vi "LIDAR Loop.vi"() -> ()   [LabVIEW 2011]
uses:
  <vilib>/Platform/TimedLoop/XDataNode/timing_clust.ctl
  <vilib>/Platform/TimedLoop/XDataNode/nitl_modes.ctl
  <vilib>/Platform/TimedLoop/XDataNode/wakeup.ctl
  <instrlib>/Hokuyo URG Series/Public/Initialize-Standard.vi
  <vilib>/Platform/TimedLoop/XDataNode/XDataNode.xnode
  <vilib>/Platform/TimedLoop/XDataNode/XDNodeRunTimeDep.lvlib
  <instrlib>/Hokuyo URG Series/Hokuyo URG Series.lvlib
panel:
  in  "maximum":dbl=300.0 format="%0.2f"
  out "Data Aquired":picture
  in  "error in":errorcluster
  in  "VISA resource name":refnum<visa-resource-name>
  in  "Debug":bool=TRUE
  out "LIDAR Data":cluster{"Magnitude":dbl[], "Direction":dbl[]}
  in  "end point (135°)":dbl=135.0
  in  "start point (-135°)":dbl=-135.0
  out "error out":errorcluster
  in  "protocol":u32(ring)=2 items=["Convert to Latest", "SCIP 1.1", "SCIP 2.0"]
  in  "stop?":bool
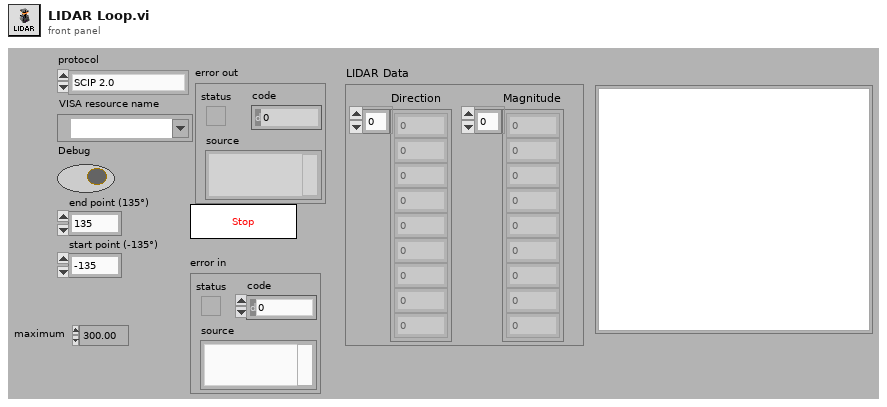
[diagram p1: front panel]
types:
  T1 = typedef "XDNodeRunTimeDep.lvlib/timing_clust.ctl" = cluster{"Expected End [f-1]":u64, "Actual End [f-1]":u64, "Finished Late? [f-1]":bool, "Expected End [i-1]":u64, "Actual End [i-1]":u64, "Finished Late? [i-1]":bool, "Expected Start [i]":u64, "Actual Start [i]":u64, "Expected Start [f]":u64, "Actual Start [f]":u64, "Source Name":string, "Structure Name":string, "Period":i64, "Deadline":i64, "Offset":i64, "Start":i64, "Priority":i32, "Timeout":i32, "Mode":T2, "Wakeup Reason":T3, "Error":errorcluster, "Source Type":string, "Secondary Source Type":string, "Global End Time":u64, "Global Start Time":u64, "Frame Duration":u64, "Iteration Duration":u64, "Assigned CPU":i32, "I/O Scan Engine Mode":u32}
  T2 = typedef "XDNodeRunTimeDep.lvlib/nitl_modes.ctl" = enum32{"No Change", "Process missed periods, maintain original phase", "Discard missed periods, maintain original phase", "Process missed periods, ignore original phase", "Discard missed periods, ignore original phase"}
  T3 = typedef "XDNodeRunTimeDep.lvlib/wakeup.ctl" = enum32{"Normal", "Aborted", "Asynchronous wakeup", "Timing source error", "Timed loop error", "Timeout"}
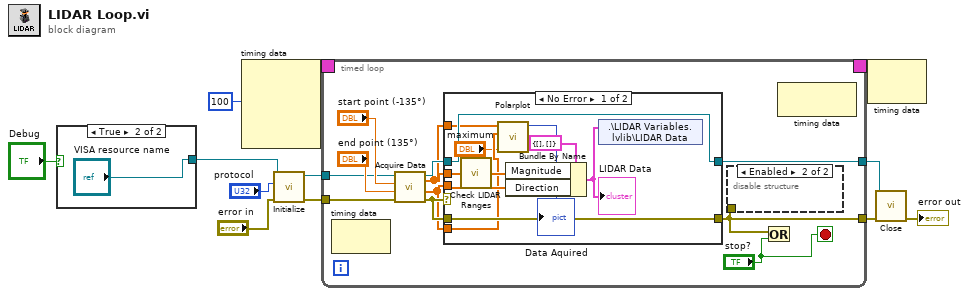
[diagram p0: block diagram]
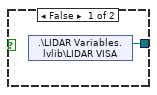
[diagram p2: hidden frame]
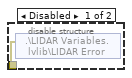
[diagram p3: hidden frame]
diagram:
  n1 = case shown="True" "Debug" {
    tunnel: [w13 "VISA resource name"] -> w6
    frame False {
      n2 = shared-variable ".\\LIDAR Variables.lvlib\\LIDAR VISA"() -> (w13:refnum<visa-resource-name>)  [unwired: 1 in, 1 out]
    }
    frame True {
    }
  }
  n3 = node-c288(i64 100 ("Period")) -> (w12:T1)  [unwired: 3 out]
  n4 = call-poly <instrlib>:"Initialize.vi"("error in (no error)"="error in", "Protocol (2: SCIP 2.0)"="protocol", "VISA resource name"=w6) -> ("error out"=w4:errorcluster, "VISA resource name out"=w5:refnum<visa-resource-name>)  [unwired: 7 in]
  n5 = timed-loop {
    timing: w12 -> [_]
    timing-out: [_] -> w11
    tunnel: w5 -> [w23]
    tunnel: [w21] -> w9
    tunnel: [w18] -> w8
    tunnel: w4 -> [w19]
    stop <- "stop?" stop-if-true
    n6 = node-c288() -> ()  [unwired: 2 out]
    n7 = call <instrlib>:"Acquire Data.vi"("error in (no error)"=w19, "End Point (120°)"="end point (135°)", "Start Point (-120°)"="start point (-135°)", "VISA resource name"=w23) -> ("error out"=w20:errorcluster, "Direction"=w15:dbl[], "Magnitude"=w16:dbl[], "VISA resource name out"=w22:refnum<visa-resource-name>)  [unwired: 4 in]
    n8 = case shown="No Error" w20 {
      selector: w20 -> [_ w38]
      tunnel: w16 -> [w31 _]
      tunnel: w15 -> [w34 _]
      tunnel: w22 -> [w37 w39]
      tunnel: [w37 w39] -> w21
      tunnel: [w36 w38] -> w18
      tunnel: w20 -> [w36 _]
      tunnel: w16 -> [w30 _]
      tunnel: w15 -> [w29 _]
      frame No Error {
        n9 = call "Check LIDAR Ranges.vi"("Magnitude"=w31) -> ("Magnitude out"=w32:dbl[])  [unwired: 4 in]
        n10 = call "Polarplot.vi"("maximum"="maximum", "Direction"=w29, "Magnitude"=w30) -> ("Data Aquired"=→"Data Aquired":picture)  [unwired: 8 in]
        n11 = Bundle By Name(cluster=cluster{"Magnitude":dbl[], "Direction":dbl[]} {"Magnitude"=[], "Direction"=[]} ("LIDAR Data"), "Magnitude"=w32, "Direction"=w34) -> (w33:cluster{"Magnitude":dbl[], "Direction":dbl[]})
        "LIDAR Data" <- w33
        n12 = shared-variable ".\\LIDAR Variables.lvlib\\LIDAR Data"(w33) -> ()  [unwired: 1 in, 1 out]
      }
      frame Error {
      }
    }
    n13 = disable-structure shown="Enabled" {
      disable-tunnel: w18 -> [w26 _]
      frame Disabled {
        n14 = shared-variable ".\\LIDAR Variables.lvlib\\LIDAR Error"(w26) -> ()  [unwired: 1 in, 1 out]
      }
      frame Enabled {
      }
    }
    n15 = Or(x=w18, y="stop?") -> ()  [unwired: 1 out]
    n16 = node-c288() -> ()  [unwired: 2 out]
  }
  n17 = node-c288(w11) -> ()  [unwired: 1 out]
  n18 = call <instrlib>:"Close.vi"("error in (no error)"=w8, "VISA resource name"=w9) -> ("error out"=→"error out":errorcluster)  [unwired: 9 in]
